vi "integrator.vi"(3 "Dt":dbl, 4 "Ic":bool, 5 "Ic_value":dbl, 6 "In":dbl) -> (0 "Out":dbl)   [LabVIEW 2023]
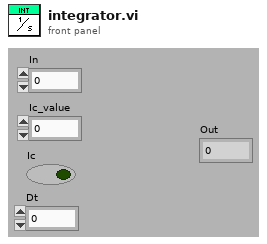
[diagram p1: front panel]
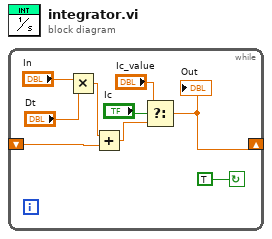
[diagram p0: block diagram]
diagram:
  n1 = while {
    shift-right: [w1] -> _
    shift-left: _ -> [w8]
    stop <- TRUE continue-if-true
    n2 = Multiply(x="In", y="Dt") -> (x*y=w5:dbl)
    n3 = Add(x=w5, y=w8) -> (x+y=w2:dbl)
    n4 = Select(t="Ic_value", s="Ic", f=w2) -> (s? t:f=w1:dbl)
    "Out" <- w1
  }
